vi "set_electrodes (SubVI).vi"(0 "Tot Electrode Arr":dbl[](array[numeric]), 5 "electrodes task 2":refnum<k21>, 9 "electrodes error":errorcluster, 11 "electrodes reference":refnum<vi>, 12 "Num samples":i32) -> (4 "electrode arr":dbl[][](array[numeric]), 6 "electrodes task":refnum<k21>, 10 "DC volts arr":dbl[](array[numeric]), 13 "Use arbitrary\nforce func?":bool, 14 "Electrode to sweep:":i32, 15 "electrodes task error":errorcluster)   [LabVIEW 2014]
uses:
  <vilib>/measure/NI_MABase.lvlib
  <resource>/objmgr/daqmx.rc
panel:
  out "SampClk.Rate":dbl
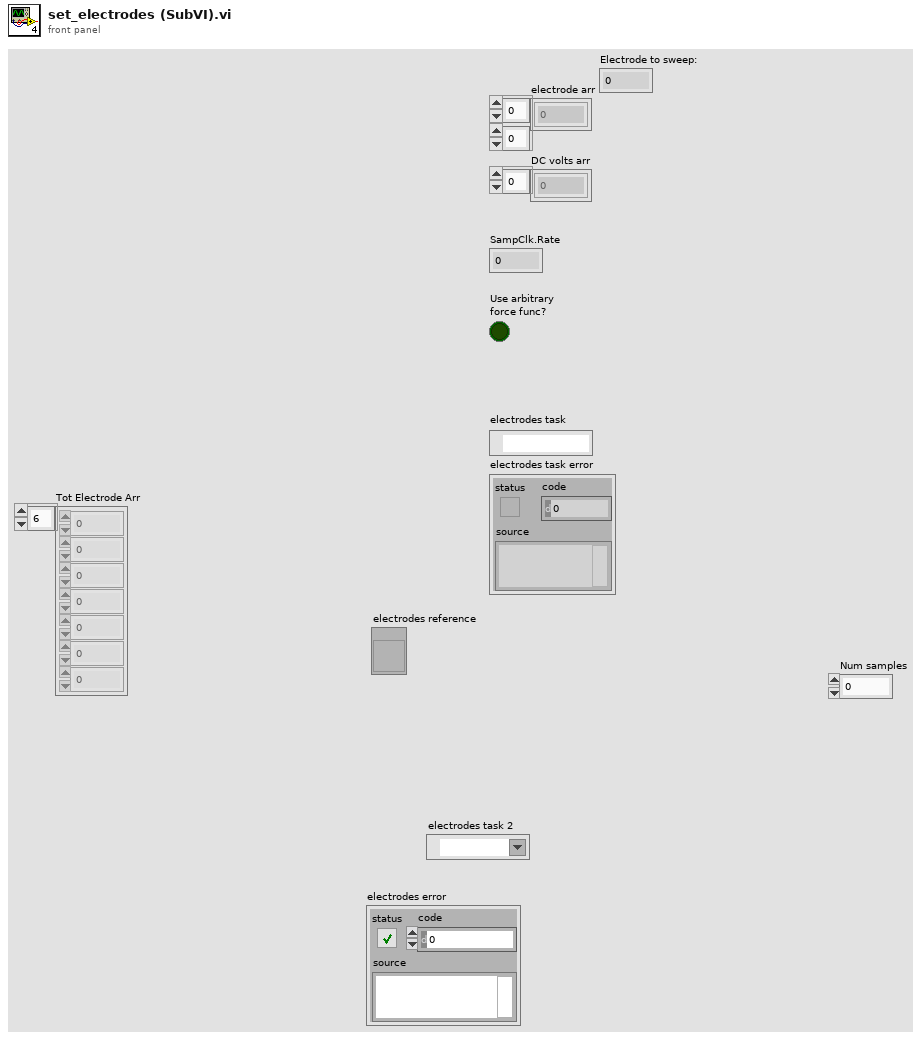
[diagram p1: front panel]
types:
  T1 = cluster{"DC volts (V):\n":dbl[], "Electrode to sweep:":i32, "start volt (V)":ext, "stop volt (V) ":ext, "# V Steps":i32, "start freq (Hz)":ext, "stop freq (Hz) ":ext, "# F steps":i32, "start DC (V)":ext, "stop DC (V)":ext, "# DC steps ":i32, "Digitize electrode\ndrives?":bool, "Sweep electrode?":bool, "Add 0.5*V DC \noffset for amp?":bool, "Use electrode \nconfig file?":bool, "Path":path, "Use arbitrary\nforce func?":bool, "Voltage vs pos file":path}
  T2 = enum16{"Sine Wave", "Triangle Wave", "Square Wave", "Sawtooth Wave"}
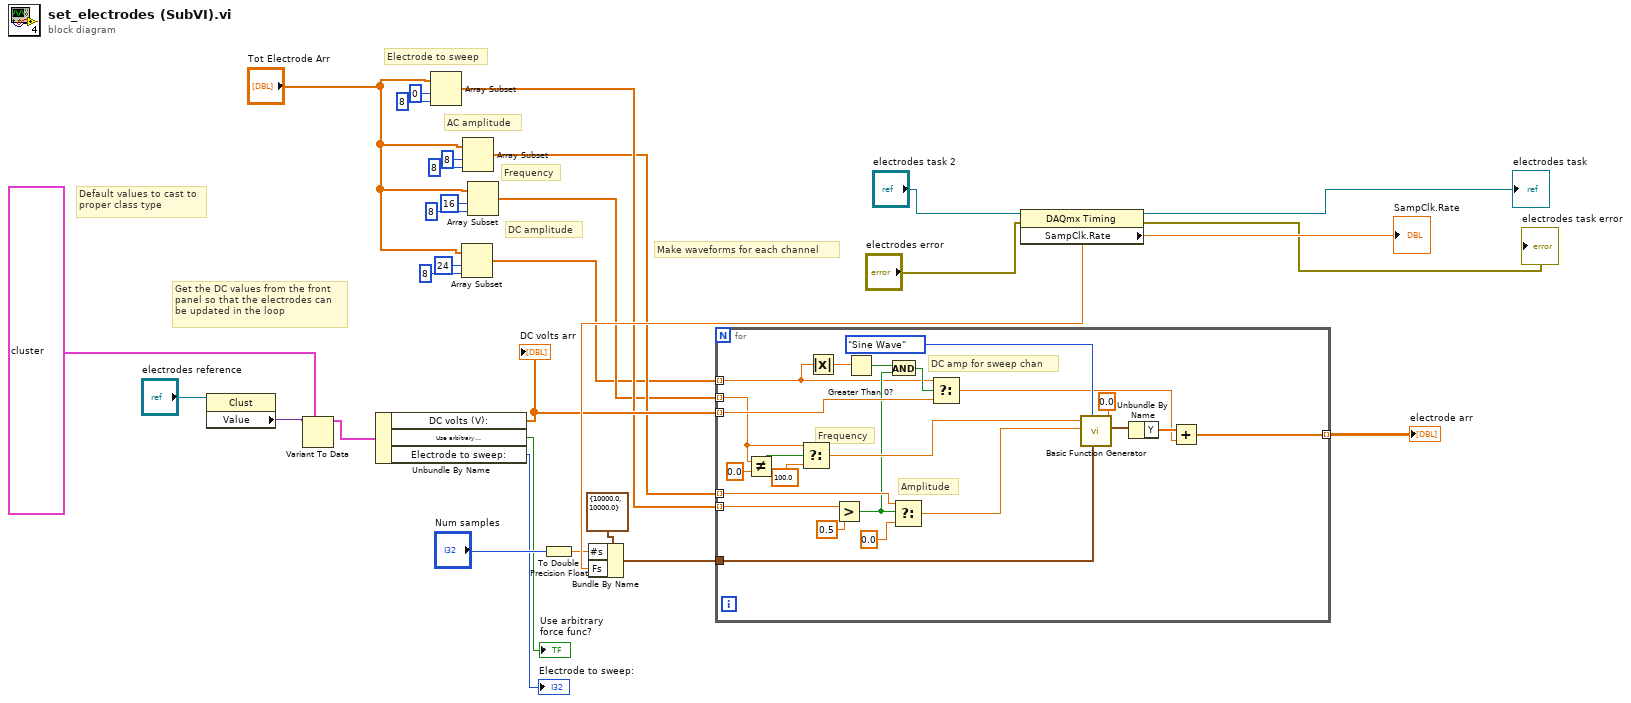
[diagram p0: block diagram]
diagram:
  # "Default values to cast to\nproper class type"
  # "Get the DC values from the front\npanel so that the electrodes can\nbe updated in the loop"
  # "Make waveforms for each channel"
  # "DC amplitude"
  # "Frequency"
  # "AC amplitude"
  # "Electrode to sweep"
  n1 = property class="Clust"(reference="electrodes reference") -> ("Value"=w21:variant)  [unwired: 1 in, 2 out]
  n2 = Variant To Data(type=T1 {"DC volts (V):\n"=[0.0, 0.0, 0.0, 0.0, 0.0, 0.0, 0.0, 0.0], "Electrode to sweep:"=3, "start volt (V)"=0.0, "stop volt (V) "=0.0, "# V Steps"=1, "start freq (Hz)"=41.0, "stop freq (Hz) "=41.0, "# F steps"=1, "start DC (V)"=0.0, "stop DC (V)"=0.0, "# DC steps "=1, "Digitize electrode\ndrives?"=TRUE, "Sweep electrode?"=FALSE, "Add 0.5*V DC \noffset for amp?"=FALSE, "Use electrode \nconfig file?"=FALSE, "Path"=path "", "Use arbitrary\nforce func?"=FALSE, "Voltage vs pos file"=path ""} ("Electrode settings:"), Variant=w21) -> (data=w20:T1)  [unwired: 1 in, 1 out]
  n3 = Unbundle By Name(w20) -> ("DC volts (V):"=w19:dbl[], "Use arbitrary\nforce func?"=→"Use arbitrary\nforce func?":bool, "Electrode to sweep:"=→"Electrode to sweep:":i32)
  "DC volts arr" <- w19
  n4 = Array Subset(array="Tot Electrode Arr", index=0, length=8) -> (w16:dbl[])
  n5 = Array Subset(array="Tot Electrode Arr", index=24, length=8) -> (w8:dbl[])
  n6 = Array Subset(array="Tot Electrode Arr", index=8, length=8) -> (w15:dbl[])
  n7 = Array Subset(array="Tot Electrode Arr", index=16, length=8) -> (w10:dbl[])
  n8 = To Double Precision Float(number="Num samples") -> (double precision float=w4:dbl)
  n9 = property class="DAQmx Timing"(reference="electrodes task 2", error in="electrodes error") -> (reference out=→"electrodes task":refnum<k21>, error out=→"electrodes task error":errorcluster, "SampClk.Rate"=w26:dbl)
  "SampClk.Rate" <- w26
  n10 = Bundle By Name(cluster=cluster{"Fs":dbl, "#s":dbl} {"Fs"=10000.0, "#s"=10000.0} ("sampling info"), "#s"=w4, "Fs"=w26) -> (w30:cluster{"Fs":dbl, "#s":dbl})
  n11 = for {
    tunnel: w19 -> [w47] mode=indexing
    tunnel: w10 -> [w42] mode=indexing
    tunnel: w15 -> [w50] mode=indexing
    tunnel: w30 -> [w49]
    tunnel: [w34] -> w25 mode=indexing
    tunnel: w8 -> [w31] mode=indexing
    tunnel: w16 -> [w46] mode=indexing
    # "DC amp for sweep chan"
    # "Frequency"
    # "Amplitude"
    n12 = Not Equal?(x=w42, y=0.0) -> (x != y?=w43:bool)
    n13 = Select(t=w42, s=w43, f=100.0) -> (s? t:f=w41:dbl)
    n14 = Absolute Value(x=w31) -> (abs(x)=w32:dbl)
    n15 = Greater?(x=w46, y=0.5) -> (0:w38:bool)
    n16 = Greater Than 0?(x=w32) -> (x > 0?=w33:bool)
    n17 = And(x=w33, y=w38) -> (x .and. y?=w39:bool)
    n18 = Select(t=w50, s=w38, f=0.0) -> (s? t:f=w52:dbl)
    n19 = Select(t=w31, s=w39, f=w47) -> (s? t:f=w35:dbl)
    n20 = call <vilib>:"Basic Function Generator.vi"("offset"=0.0, "sampling info"=w49, "signal type"=T2."Sine Wave", "amplitude"=w52, "frequency"=w41) -> ("signal out"=w48:waveform(dbl))  [unwired: 4 in, 2 out]
    n21 = Unbundle By Name(w48) -> ("Y"=w36:dbl[])
    n22 = Add(x=w36, y=w35) -> (x+y=w34:dbl[])
  }
  "electrode arr" <- w25
